vi "Initialize.vi"(8 "error in (no error)":errorcluster, 11 "device data model in":refnum<class "Standard Data Model.lvclass">) -> (0 "error out":errorcluster, 3 "device data model out":refnum<class "Standard Data Model.lvclass">)   [LabVIEW 2017, in "SubVIs.lvlib" / "Standard Data Model.lvclass"]
doc: "This VI initializes the device data model."
uses:
  <vilib>/Modbus/subvis/Data and Functions/Standard Data Model/Standard Data Model.lvclass
  <vilib>/Modbus/subvis/Data and Functions/Standard Data Model/Standard Data Model.lvclass/Standard Data Model.ctl
  <vilib>/Modbus/subvis/Data and Functions/Device Data Model/Device Data Model.lvclass
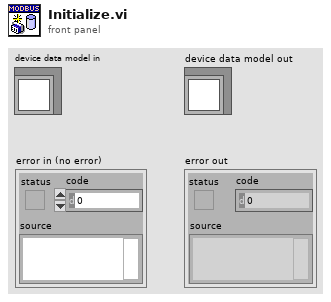
[diagram p1: front panel]
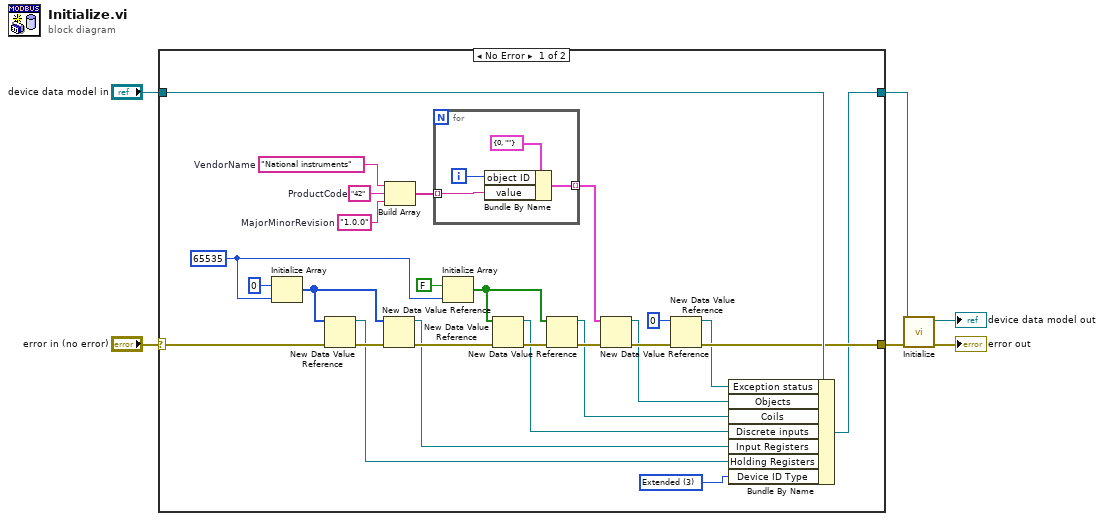
[diagram p0: block diagram]
diagram:
  n1 = case shown="No Error" "error in (no error)" {
    selector: "error in (no error)" -> [w7 w38]
    tunnel: "device data model in" -> [w27 w39]
    tunnel: [w16 w38] -> w5
    tunnel: [w15 w39] -> w4
    frame No Error {
      w9 = u8 3 items=["Basic"=1, "Regular "=2, "Extended"=3] ("Read Device ID Code")
      w28 = "1.0.0"  # MajorMinorRevision
      w30 = "42"  # ProductCode
      w29 = "National instruments"  # VendorName
      w31 = u16 65535
      n2 = Initialize Array(u16 0 ("Numeric"), w31) -> (w21:u16[])
      n3 = New Data Value Reference(data value=w21, error in=w7) -> (data value reference=w14:refnum<data-value>, error out=w23:errorcluster)
      n4 = New Data Value Reference(data value=w21, error in=w23) -> (data value reference=w13:refnum<data-value>, error out=w24:errorcluster)
      n5 = Build Array(w29, w30, w28) -> (w26:string[])
      n6 = for {
        tunnel: w26 -> [w35] mode=indexing
        tunnel: [w34] -> w20 mode=indexing
        i -> [w36]
        n7 = Bundle By Name(cluster=cluster{"object ID":u8, "value":string} {"object ID"=0, "value"=""} ("Cluster"), "object ID"=w36, "value"=w35) -> (w34:cluster{"object ID":u8, "value":string})
      }
      n8 = Initialize Array(FALSE ("Boolean"), w31) -> (w22:bool[])
      n9 = New Data Value Reference(data value=w22, error in=w24) -> (data value reference=w12:refnum<data-value>, error out=w25:errorcluster)
      n10 = New Data Value Reference(data value=w22, error in=w25) -> (data value reference=w11:refnum<data-value>, error out=w19:errorcluster)
      n11 = New Data Value Reference(data value=w20, error in=w19) -> (data value reference=w10:refnum<data-value>, error out=w18:errorcluster)
      n12 = New Data Value Reference(data value=u8 0, error in=w18) -> (data value reference=w8:refnum<data-value>, error out=w16:errorcluster)
      n13 = Bundle By Name(cluster=w27, "Exception status"=w8, "Objects"=w10, "Coils"=w11, "Discrete inputs"=w12, "Input Registers"=w13, "Holding Registers"=w14, "Device ID Type"=w9) -> (w15:refnum<class "Standard Data Model.lvclass">)
    }
    frame Error {
    }
  }
  n14 = call-parent "Initialize.vi"("error in (no error)"=w5, "device data model in"=w4) -> ("error out"=→"error out":errorcluster, "device data model out"=→"device data model out":refnum<class "Standard Data Model.lvclass">)  [unwired: 8 in]
